vi "UltrasonicStopping.vi"(0 "SonarMB1010AnalogDevRef":T1={"AIDeviceRef"={"DevStatus"={"status"=FALSE, "code"=0, "source"=""}, "Analog Channel"=enum."Invalid"}, "Scaling factor (V/in)"=0.0098, "Average Bits"=3} {"Average Bits" max=15}, 1 "SonarMB1010AnalogDevRef 2":T1={"AIDeviceRef"={"DevStatus"={"status"=FALSE, "code"=0, "source"=""}, "Analog Channel"=enum."Invalid"}, "Scaling factor (V/in)"=0.0098, "Average Bits"=3} {"Average Bits" max=15}, 2 "X":dbl, 3 "Y":dbl, 4 "Dist(in.)":dbl) -> (5 "X":dbl, 6 "Y":dbl)   [LabVIEW 2017]
uses:
  <vilib>/Rock Robotics/WPI/Ultrasonic/WPI_SonarMB1010AnalogDeviceRef.ctl
  <vilib>/Rock Robotics/WPI/AnalogChannel/WPI_AnalogChannelDevRef.ctl
  <vilib>/Rock Robotics/SystemInterfaces/AI/FPGA_AIChannel.ctl
  <vilib>/Rock Robotics/WPI/Ultrasonic/WPI_SonarMB1010AnalogGetRange.vi
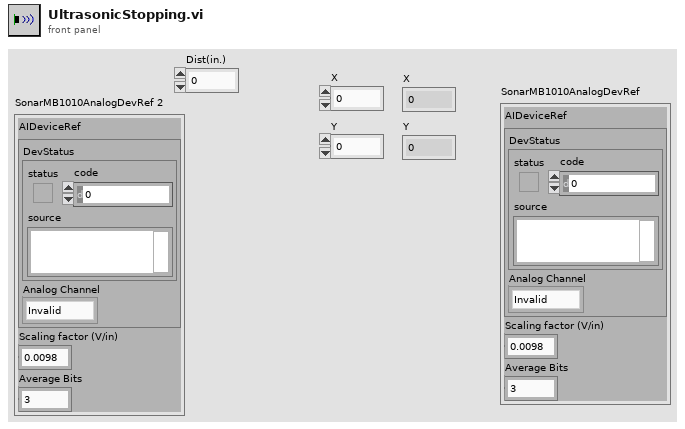
[diagram p1: front panel]
types:
  T1 = typedef "WPI_SonarMB1010AnalogDeviceRef.ctl" = cluster{"AIDeviceRef":T2, "Scaling factor (V/in)":dbl, "Average Bits":u8}
  T2 = typedef "WPI_AnalogChannelDevRef.ctl" = cluster{"DevStatus":errorcluster, "Analog Channel":T3}
  T3 = typedef "FPGA_AIChannel.ctl" = enum8{"AI 0", "AI 1", "AI 2", "AI 3", "AI MXP 0", "AI MXP 1", "AI MXP 2", "AI MXP 3", "Invalid"}
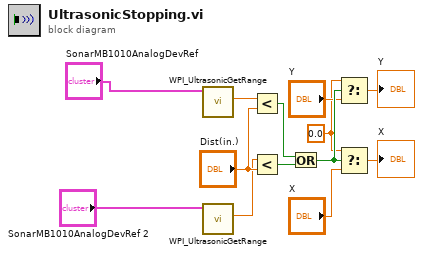
[diagram p0: block diagram]
diagram:
  w3 = 0.0
  n1 = call-poly <vilib>:"WPI_UltrasonicGetRange.vi"("SonarMB1010AnalogDevRef"="SonarMB1010AnalogDevRef") -> ("Distance"=w12:dbl)  [unwired: 8 in, 2 out]
  n2 = call-poly <vilib>:"WPI_UltrasonicGetRange.vi"("SonarMB1010AnalogDevRef"="SonarMB1010AnalogDevRef 2") -> ("Distance"=w11:dbl)  [unwired: 8 in, 2 out]
  n3 = Less?(x=w12, y="Dist(in.)") -> (x < y?=w10:bool)
  n4 = Less?(x=w11, y="Dist(in.)") -> (x < y?=w9:bool)
  n5 = Or(x=w10, y=w9) -> (x .or. y?=w8:bool)
  n6 = Select(t=w3, s=w8, f="Y") -> (s? t:f=→"Y":dbl)
  n7 = Select(t=w3, s=w8, f="X") -> (s? t:f=→"X":dbl)
